vi "OpenVINO_ONNX_DEMO.vi"() -> ()   [LabVIEW 2020]
uses:
  LVOpenVINO.dll
panel:
  out "result":T1(array[cluster])
  out "Image":T2(plugin-control)
  out "return type":i32
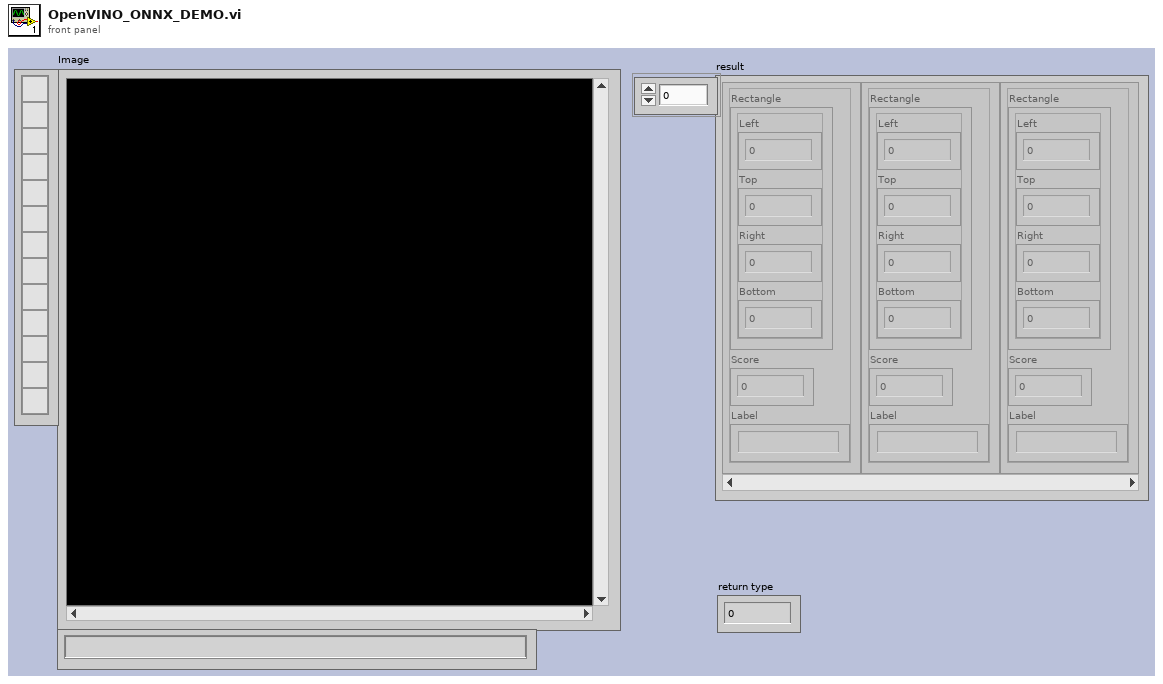
[diagram p1: front panel]
types:
  T1 = cluster{"Rectangle":cluster{"Left":i32, "Top":i32, "Right":i32, "Bottom":i32}, "Score":sgl, "Label":string}[]
  T2 = typedef "IMAQ Image.ctl" = refnum<image>
  T3 = typedef "Image Type" = u32
  T4 = cluster{"Left":i32, "Top":i32, "Right":i32, "Bottom":i32}
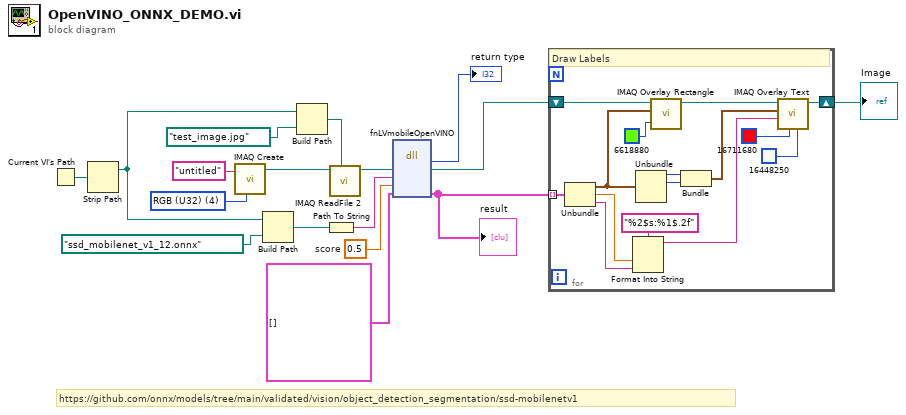
[diagram p0: block diagram]
diagram:
  w3 = sgl 0.5  # score
  w15 = T3 4 items=["Grayscale (U8)", "Grayscale (I16)", "Grayscale (SGL)", "Complex (CSG)", "RGB (U32)", "HSL (U32)", "RGB (U64)", "Grayscale (U16)"] ("Image Type")
  # "https://github.com/onnx/models/tree/main/validated/vision/object_detection_segmentation/ssd-mobilenetv1"
  n1 = Current VI's Path() -> (path=w8:path)
  n2 = Strip Path(path=w8) -> (stripped path=w1:path)  [unwired: 1 out]
  n3 = call "IMAQ Create"("Image Name"="untitled", "Image Type"=w15) -> ("New Image"=w14:T2)  [unwired: 3 in, 1 out]
  n4 = Build Path(base path=w1, name or relative path=path "ssd_mobilenet_v1_12.onnx") -> (appended path=w6:path)
  n5 = Build Path(base path=w1, name or relative path=path "test_image.jpg") -> (appended path=w4:path)
  n6 = Path To String(path=w6) -> (string=w10:string)
  n7 = call "IMAQ ReadFile 2"("File Path"=w4, "Image"=w14) -> ("Image Out"=w2:T2)  [unwired: 5 in, 4 out]
  n8 = dll-call lib="D:/ssd-mobilenet-labview/LabVIEW-Example/LVOpenVINO.dll" fn="fnLVmobileOpenVINO"("src"=w2, "model"=w10, "score"=w3, "result"=T1 []) -> ("return type"=→"return type":i32, "src"=w12:T2, "result"=w9:T1)  [unwired: 5 in, 2 out]
  "result" <- w9
  n9 = for {
    shift-right: [w27] -> w11
    shift-left: w12 -> [w32]
    tunnel: w9 -> [w31] mode=indexing
    # "Draw Labels"
    n10 = Unbundle(w31) -> ("Rectangle"=w26:T4, "Score"=w20:sgl, "Label"=w19:string)
    n11 = Format Into String(format string="%2$s:%1$.2f", w20, w19) -> (resulting string=w22:string)  [unwired: 2 in, 1 out]
    n12 = Unbundle(w26) -> ("Left"=w25:i32, "Top"=w24:i32)  [unwired: 2 out]
    n13 = call "IMAQ Overlay Rectangle"("Color"=u32 6618880, "Rectangle"=w26, "Image"=w32) -> ("Image Out"=w28:T2)  [unwired: 7 in, 1 out]
    n14 = Bundle("Left"=w25, "Top"=w24) -> (w23:cluster{"Left":i32, "Top":i32})  [unwired: 1 in]
    n15 = call "IMAQ Overlay Text"("BG Color (Transparent)"=u32 16448250, "Text Color (black)"=u32 16711680, "String"=w22, "Origin"=w23, "Image"=w28) -> ("Image Out"=w27:T2)  [unwired: 5 in, 1 out]
  }
  "Image" <- w11
